vi "Query Float.vi"(8 "error in (no error)":errorcluster, 10 "write buffer":string, 11 "VISA resource name In":refnum<visa-resource-name>) -> (0 "error out":errorcluster, 2 "float":dbl, 3 "VISA resource name out":refnum<visa-resource-name>)   [LabVIEW 2013, in "Newport 1830-C.lvlib"]
doc: "Reads a float from the output buffer of the instrument."
uses:
  Newport 1830-C.lvlib
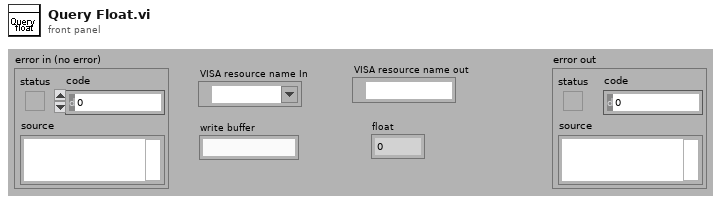
[diagram p1: front panel]
types:
  T1 = typedef "Semaphore RefNum" = refnum<k1>
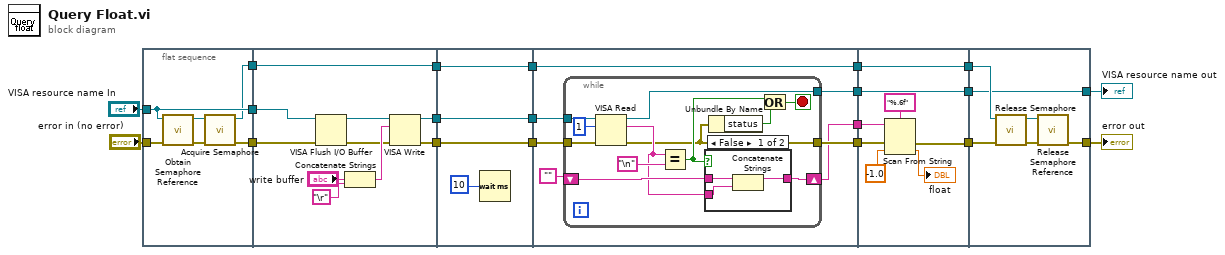
[diagram p0: block diagram]
diagram:
  n1 = flat-sequence {
    tunnel: "VISA resource name In" -> [w23]
    tunnel: "error in (no error)" -> [w26]
    tunnel: [w23] -> w18
    tunnel: [w22] -> w17
    tunnel: [w21] -> w9
    tunnel: w18 -> [w28]
    tunnel: w17 -> [w27]
    tunnel: [w36] -> w15
    tunnel: [w35] -> w13
    tunnel: [w34] -> w10
    tunnel: w9 -> [w34]
    tunnel: [w39] -> w16
    tunnel: w15 -> [w39]
    tunnel: [w38] -> w14
    tunnel: w13 -> [w38]
    tunnel: [w37] -> w11
    tunnel: w10 -> [w37]
    tunnel: w16 -> [w46]
    tunnel: w14 -> [w45]
    tunnel: [w47] -> w7
    tunnel: w11 -> [w47]
    tunnel: [w44] -> w5
    tunnel: [w42] -> w4
    tunnel: [w41] -> w2
    tunnel: [w68] -> w8
    tunnel: w7 -> [w71]
    tunnel: [w71] -> w6
    tunnel: w5 -> [w67]
    tunnel: w4 -> [w66]
    tunnel: w2 -> [w64]
    tunnel: [w64] -> w1
    tunnel: w8 -> [w77]
    tunnel: [w75] -> w12
    tunnel: w6 -> [w74]
    tunnel: [w72] -> w3
    tunnel: w1 -> [w72]
    frame #0 {
      n2 = call <vilib>:"Obtain Semaphore Reference.vi"("error in (no error)"=w26, "name (unnamed)"=w23) -> ("error out"=w25:errorcluster, "semaphore"=w24:T1)  [unwired: 3 in, 1 out]
      n3 = call <vilib>:"Acquire Semaphore.vi"("error in (no error)"=w25, "semaphore"=w24) -> ("error out"=w22:errorcluster, "semaphore out"=w21:T1)  [unwired: 3 in, 1 out]
    }
    frame #1 {
      n4 = VISA Flush I/O Buffer(VISA resource name=w28, error in (no error)=w27) -> (VISA resource name out=w29:refnum<visa-resource-name>, error out=w30:errorcluster)  [unwired: 1 in]
      n5 = Concatenate Strings("write buffer", "\r") -> (w31:string)
      n6 = VISA Write(VISA resource name=w29, write buffer=w31, error in (no error)=w30) -> (VISA resource name out=w36:refnum<visa-resource-name>, error out=w35:errorcluster)  [unwired: 1 out]
    }
    frame #2 {
      n7 = Wait (ms)(milliseconds to wait=u32 10) -> ()  [unwired: 1 out]
    }
    frame #3 {
      n8 = while {
        tunnel: w46 -> [w59]
        tunnel: w45 -> [w58]
        tunnel: [w48] -> w44
        shift-right: [w54] -> w42
        shift-left: "" -> [w55]
        tunnel: [w52] -> w41
        stop <- w51 stop-if-true
        n9 = VISA Read(VISA resource name=w59, byte count=u32 1, error in (no error)=w58) -> (VISA resource name out=w52:refnum<visa-resource-name>, read buffer=w53:string, error out=w48:errorcluster)  [unwired: 1 out]
        n10 = Equal?(x=w53, y="\n") -> (x = y?=w50:bool)
        n11 = case shown="False" w50 {
          tunnel: [w62 w63] -> w54
          tunnel: w55 -> [w61 w63]
          tunnel: w53 -> [w60 _]
          frame False {
            n12 = Concatenate Strings(w61, w60) -> (w62:string)
          }
          frame True {
          }
        }
        n13 = Unbundle By Name(w48) -> ("status"=w49:bool)
        n14 = Or(x=w50, y=w49) -> (x .or. y?=w51:bool)
      }
    }
    frame #4 {
      n15 = Scan From String(format string="%.6f", input string=w66, error in=w67, default 1=-1.0 ("default value 1")) -> (error out=w68:errorcluster, output 1=→"float":dbl)  [unwired: 1 in, 2 out]
    }
    frame #5 {
      n16 = call <vilib>:"Release Semaphore.vi"("error in (no error)"=w77, "semaphore"=w74) -> ("error out"=w76:errorcluster, "semaphore out"=w73:T1)  [unwired: 4 in]
      n17 = call <vilib>:"Release Semaphore Reference.vi"("error in (no error)"=w76, "semaphore"=w73) -> ("error out"=w75:errorcluster)  [unwired: 8 in, 1 out]
    }
  }
  "error out" <- w12
  "VISA resource name out" <- w3
